vi "Find.vi"(8 "error in (no error)":errorcluster, 11 "Configurations":refnum<class "Configuration.lvclass">[](array[class])) -> (0 "error out":errorcluster, 1 "found?":bool, 2 "index":i32, 3 "Core Framework Configuration":refnum<class "Core Framework Configuration.lvclass">)   [LabVIEW 2017, in "DSF Core.lvlib" / "Core Framework Configuration.lvclass"]
uses:
  Core Framework Configuration.lvclass
  Configuration.lvclass
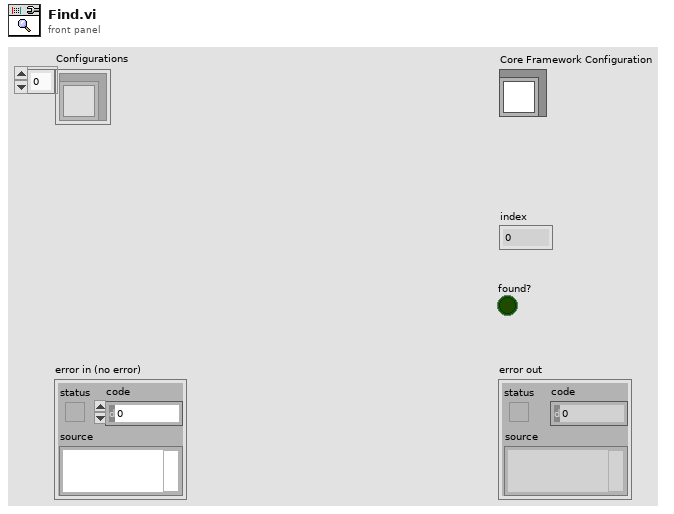
[diagram p1: front panel]
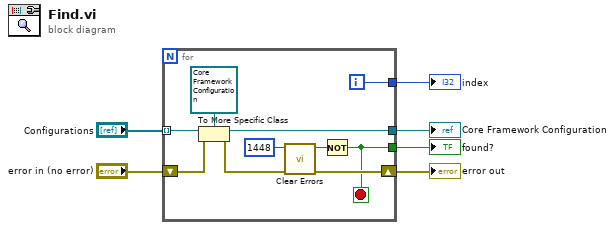
[diagram p0: block diagram]
diagram:
  n1 = for {
    tunnel: "Configurations" -> [w16] mode=indexing
    shift-right: [w13] -> w3
    shift-left: "error in (no error)" -> [w12]
    tunnel: [w10] -> w2
    tunnel: [w9] -> w4
    tunnel: [w7] -> w1
    i -> [w7]
    stop <- w10 stop-if-true
    n2 = To More Specific Class(target class=refnum<class "Core Framework Configuration.lvclass"> refnum ("Core Framework Configuration out"), reference=w16, error in=w12) -> (specific class reference=w9:refnum<class "Core Framework Configuration.lvclass">, error out=w14:errorcluster)
    n3 = call <vilib>:"Clear Errors.vi"("error in (no error)"=w14, "specific error code to clear (0: all)"=1448) -> ("error out"=w13:errorcluster, "specific error cleared?"=w11:bool)  [unwired: 4 in]
    n4 = Not(x=w11) -> (.not. x?=w10:bool)
  }
  "error out" <- w3
  "Core Framework Configuration" <- w4
  "found?" <- w2
  "index" <- w1
